vi "spin.vi"(1 "Interval":dbl, 2 "relative seconds":dbl) -> (0 "relative seconds 2":dbl)   [LabVIEW 2018, in "Synchronization Device.lvlib" / "Synchronization Device.lvclass"]
uses:
  Synchronization Device.lvclass
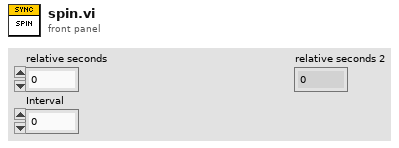
[diagram p1: front panel]
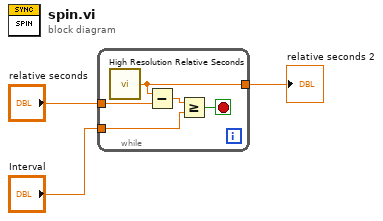
[diagram p0: block diagram]
diagram:
  n1 = while {
    tunnel: [w8] -> w1
    tunnel: "relative seconds" -> [w7]
    tunnel: "Interval" -> [w5]
    stop <- w4 stop-if-true
    n2 = call <vilib>:"High Resolution Relative Seconds.vi"() -> ("relative seconds"=w8:dbl)
    n3 = Subtract(x=w8, y=w7) -> (x-y=w6:dbl)
    n4 = Greater Or Equal?(x=w6, y=w5) -> (x >= y?=w4:bool)
  }
  "relative seconds 2" <- w1
